vi "WriteToFile.vi"(0 "convert eol? (no:F)":bool, 5 "append to file? (new file:F)":bool, 7 "advisory dialog? (display:T)":bool, 8 "character string":string, 10 "file path (dialog if empty)":path) -> (3 "new file path (Not A Path if cancelled)":path)   [LabVIEW 2014, in "Panels.lvlib"]
doc: "Writes a <B>character string</B> to a new byte stream file or appends the string to an existing file. The VI opens or creates the file before writing to it and closes it afterwards."
uses:
  Panels.lvlib
panel:
  in  "prompt":string="Choose file to write."
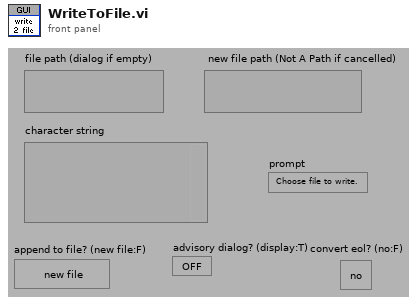
[diagram p1: front panel]
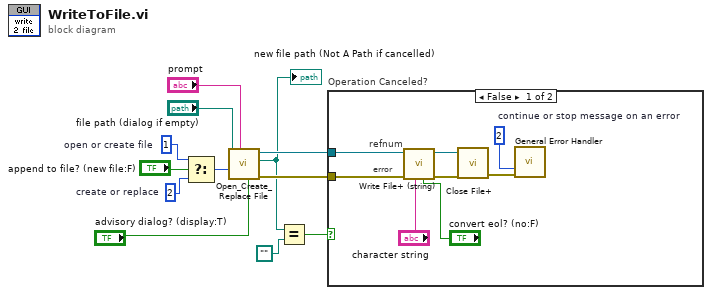
[diagram p0: block diagram]
diagram:
  w7 = i16 2  # create or replace
  w9 = i16 1  # open or create file
  n1 = Select(t=w9, s="append to file? (new file:F)", f=w7) -> (s? t:f=w10:i16)
  n2 = call <vilib>:"Open_Create_Replace File.vi"("advisory dialog? (display:T)"="advisory dialog? (display:T)", "prompt"="prompt", "function (open:0)"=w10, "file path"="file path (dialog if empty)") -> ("error out"=w11:errorcluster, "new file path"=w2:path, "refnum"=w6:refnum<file>)  [unwired: 4 in, 1 out]
  "new file path (Not A Path if cancelled)" <- w2
  n3 = Equal?(x=w2, y=path "") -> (x = y?=w1:bool)
  n4 = case "Operation Canceled?" shown="False" w1 {
    tunnel: w11 -> [w20 _]
    tunnel: w6 -> [w14 _]
    frame False {
      w19 = 2  # continue or stop message on an error
      # "error"
      # "refnum"
      n5 = call <vilib>:"Write File+ (string).vi"("convert eol? (no:F)"="convert eol? (no:F)", "string"="character string", "error in (no error)"=w20, "refnum"=w14) -> ("error out"=w18:errorcluster, "dup refnum"=w17:refnum<file>)  [unwired: 3 in, 1 out]
      n6 = call <vilib>:"Close File+.vi"("error in (no error)"=w18, "refnum"=w17) -> ("error out"=w16:errorcluster)  [unwired: 3 in, 2 out]
      n7 = call <vilib>:"General Error Handler.vi"("type of dialog (OK msg:1)"=w19, "error in (no error)"=w16) -> ()  [unwired: 9 in, 5 out]
    }
    frame True {
    }
  }
